vi "Duplicated Test Channel.vi"(6 "Test Channel File Path":path, 10 "Item Configurations":refnum<class "Item Configuration.lvclass">[](array[class]), 11 "Test Channel Directory Path":path) -> (3 "Duplicated?":bool)   [LabVIEW 2013, in "File IO.lvlib"]
uses:
  File IO.lvlib
  Item Configuration/Item Configuration/Item Configuration.lvclass
  <vilib>/xml/Load XML File.vi
  <vilib>/xml/Close Reference(Node).vi
  <vilib>/xml/NI_XML.lvlib
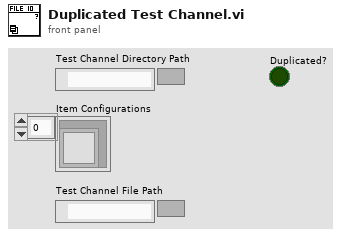
[diagram p1: front panel]
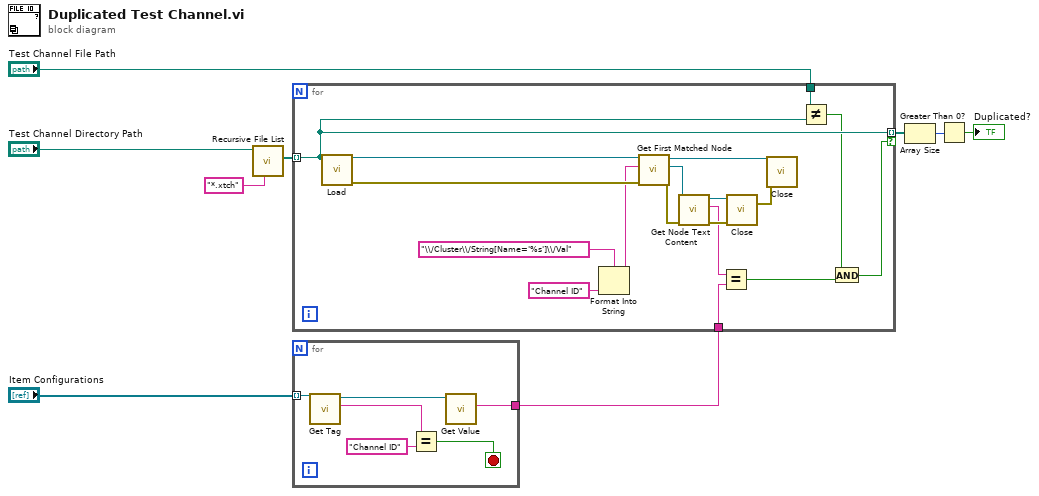
[diagram p0: block diagram]
diagram:
  n1 = call <vilib>:"Recursive File List.vi"("pattern"="*.xtch", "Folder Path"="Test Channel Directory Path") -> ("All Files in Dir"=w9:path[])  [unwired: 5 in, 4 out]
  n2 = for {
    tunnel: "Item Configurations" -> [w15] mode=indexing
    tunnel: [w10] -> w5
    stop <- w11 stop-if-true
    n3 = call-dynamic "Get Tag.vi"("Item Configuration in"=w15) -> ("Project Info Tag"=w13:string, "Item Configuration out"=w14:refnum<class "Item Configuration.lvclass">)  [unwired: 8 in, 1 out]
    n4 = Equal?(x=w13, y="Channel ID") -> (x = y?=w11:bool)
    n5 = call-dynamic "Get Value.vi"("Item Configuration in"=w14) -> ("Project Info Value"=w10:string)  [unwired: 8 in, 2 out]
  }
  n6 = for {
    tunnel: w9 -> [w19] mode=indexing
    tunnel: w5 -> [w21]
    tunnel: [w19] -> w4 mode=indexing if=w17
    tunnel: "Test Channel File Path" -> [w18]
    n7 = call-poly <vilib>:"Load.vi"("path to XML document"=w19) -> ("DOM document out"=w33:refnum<k20>, "error out"=w32:errorcluster)  [unwired: 12 in, 1 out]
    n8 = Format Into String(format string="\\/Cluster\\/String[Name='%s']\\/Val" ("XPath expression"), "Channel ID" ("input 1")) -> (resulting string=w29:string)  [unwired: 2 in, 1 out]
    n9 = call <vilib>:"Get First Matched Node.vi"("error in (no error)"=w32, "XPath expression"=w29, "node in"=w33) -> ("error out"=w27:errorcluster, "node result"=w28:refnum<k20>, "node out"=w31:refnum<k20>)  [unwired: 6 in]
    n10 = call <vilib>:"Get Node Text Content.vi"("error in (no error)"=w27, "node in"=w28) -> ("error out"=w25:errorcluster, "node text"=w22:string, "node out"=w26:refnum<k20>)  [unwired: 7 in]
    n11 = Equal?(x=w22, y=w21) -> (x = y?=w20:bool)
    n12 = call-poly <vilib>:"Close.vi"("error in (no error)"=w25, "node"=w26) -> ("error out"=w24:errorcluster)  [unwired: 7 in]
    n13 = call-poly <vilib>:"Close.vi"("error in (no error)"=w24, "node"=w31) -> ()  [unwired: 7 in, 1 out]
    n14 = Not Equal?(x=w18, y=w19) -> (x != y?=w16:bool)
    n15 = And(x=w16, y=w20) -> (x .and. y?=w17:bool)
  }
  n16 = Array Size(array=w4) -> (size(s)=w3:i32)
  n17 = Greater Than 0?(x=w3) -> (x > 0?=→"Duplicated?":bool)
